vi "Actor Core.vi"(8 "error in":errorcluster, 11 "Modbus in":refnum<class "Modbus.lvclass">) -> (0 "error out":errorcluster, 3 "Actor out":refnum<class "Actor.lvclass">)   [LabVIEW 2020, in "Modbus.lvlib" / "Modbus.lvclass"]
doc: "(<B>Filename</B>: Actor Framework.lvlib:Actor.lvclass:Actor Core.vi)\n\nReceives messages to the actor, reacts to them, and initiates any error handling that may shut the actor down.\n\nDescendant classes may override this VI to append parallel tasks for the actor to complete while it handles messages. Overrides use the Call Parent Class Method node."
uses:
  Modbus.lvclass
  F:/LV projects/Igas-Tester/Sensor/Sensor/Sensor.lvclass
  <vilib>/ActorFramework/Actor/Actor.lvclass
  Modbus.lvclass/Modbus.ctl
  Sensor/Sensor/Sensor.lvclass
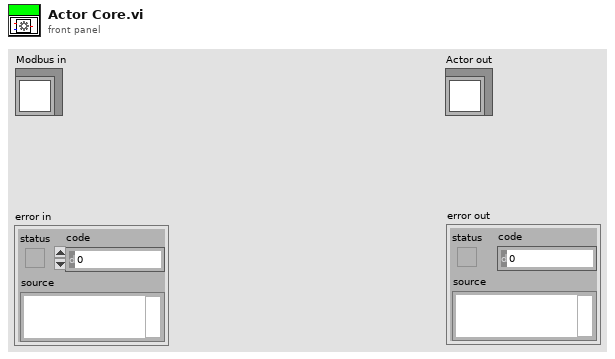
[diagram p1: front panel]
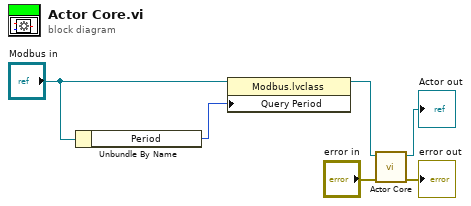
[diagram p0: block diagram]
diagram:
  n1 = Unbundle By Name("Modbus in") -> ("Period"=w2:u16)
  n2 = property class="Modbus.lvclass"(reference="Modbus in", "Query Period"=w2) -> (reference out=w4:refnum<class "Modbus.lvclass">)  [unwired: 1 in, 1 out]
  n3 = call-parent "Actor Core.vi"("error in"="error in", "Sensor in"=w4) -> ("error out"=→"error out":errorcluster, "Actor out"=→"Actor out":refnum<class "Actor.lvclass">)  [unwired: 8 in]
